vi "Generate SystemLink Software Tab shortcut.vi"() -> ()   [LabVIEW 2017]
uses:
  <vilib>/Utility/sysdir.llb/System Directory Type.ctl
panel:
  out "error out":errorcluster
  out "server URL":string
  out "local system minion ID":string
  # "Run this VI (or corresponding built EXE) to generate a Desktop shortcut to the Local System's SystemLink Software tab. \n\nNote: Before running this VI (or EXE), make sure that the local system has already successfully connected to and been approved by a SystemLink Server."
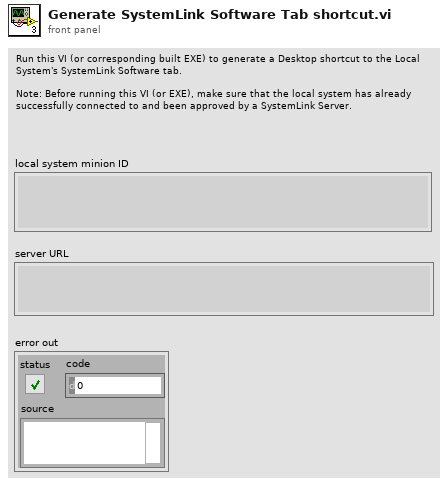
[diagram p1: front panel]
types:
  T1 = enum16{"open", "replace", "create", "open or create", "replace or create", "replace or create with confirmation"}
  T2 = typedef "System Directory Type.ctl" = i32
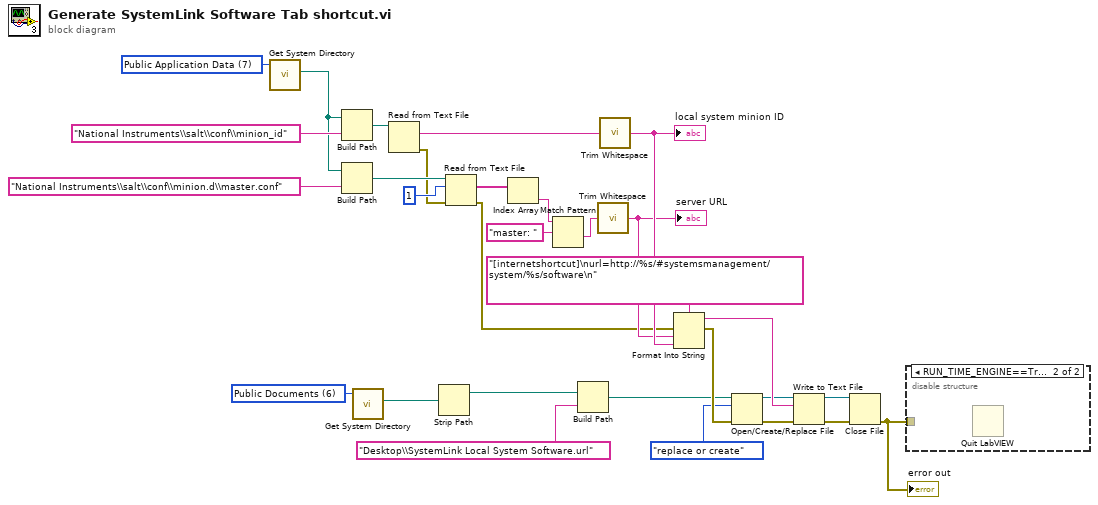
[diagram p0: block diagram]
diagram:
  w26 = T2 7 items=["User Home"=0, "User Desktop"=1, "User Documents"=2, "User Application Data"=3, "User Preferences"=4, "User Temporary"=5, "Public Documents"=6, "Public Application Data"=7, "Public Preferences"=8, "Public Cache"=13, "System Core Libraries"=9, "System Installed Libraries"=10, "Application Files"=11, "Boot Volume Root"=12] ("system directory type")
  w30 = T2 6 items=["User Home"=0, "User Desktop"=1, "User Documents"=2, "User Application Data"=3, "User Preferences"=4, "User Temporary"=5, "Public Documents"=6, "Public Application Data"=7, "Public Preferences"=8, "Public Cache"=13, "System Core Libraries"=9, "System Installed Libraries"=10, "Application Files"=11, "Boot Volume Root"=12] ("system directory type")
  n1 = call <vilib>:"Get System Directory.vi"("system directory type"=w26) -> ("system directory"=w21:path)  [unwired: 10 in]
  n2 = Build Path(base path=w21, name or relative path="National Instruments\\salt\\conf\\minion_id") -> (appended path=w24:path)
  n3 = Build Path(base path=w21, name or relative path="National Instruments\\salt\\conf\\minion.d\\master.conf") -> (appended path=w20:path)
  n4 = call <vilib>:"Get System Directory.vi"("system directory type"=w30) -> ("system directory"=w29:path)  [unwired: 10 in]
  n5 = Read from Text File(file (use dialog)=w24) -> (text=w23:string, error out=w7:errorcluster)  [unwired: 3 in, 2 out]
  n6 = Strip Path(path=w29) -> (stripped path=w28:path)  [unwired: 1 out]
  n7 = Read from Text File(file (use dialog)=w20, count=1, error in=w7) -> (text=w17:string[], error out=w6:errorcluster)  [unwired: 1 in, 2 out]
  n8 = Index Array(array=w17) -> (element=w16:string)  [unwired: 1 in]
  n9 = Match Pattern(string=w16, regular expression="master: ") -> (after substring=w14:string)  [unwired: 1 in, 3 out]
  n10 = Build Path(base path=w28, name or relative path="Desktop\\SystemLink Local System Software.url") -> (appended path=w3:path)
  n11 = call <vilib>:"Trim Whitespace.vi"("string"=w14) -> ("trimmed string"=w13:string)  [unwired: 1 in]
  "server URL" <- w13
  n12 = call <vilib>:"Trim Whitespace.vi"("string"=w23) -> ("trimmed string"=w19:string)  [unwired: 1 in]
  "local system minion ID" <- w19
  n13 = Format Into String(format string="[internetshortcut]\nurl=http://%s/#systemsmanagement/system/%s/software\n" ("name or relative path"), error in=w6, w13, w19) -> (resulting string=w11:string, error out=w5:errorcluster)  [unwired: 1 in]
  n14 = Open/Create/Replace File(file path (use dialog)=w3, error in=w5, operation (0:open)=T1."replace or create") -> (refnum out=w2:refnum<file>, error out=w4:errorcluster)  [unwired: 3 in, 1 out]
  n15 = Write to Text File(file (use dialog)=w2, text=w11, error in=w4) -> (refnum out=w10:refnum<file>, error out=w9:errorcluster)  [unwired: 1 in, 1 out]
  n16 = Close File(refnum=w10, error in=w9) -> (error out=w8:errorcluster)  [unwired: 1 out]
  "error out" <- w8
  n17 = disable-structure shown="RUN_TIME_ENGINE==True" {
    disable-tunnel: w8 -> [_ _]
    frame condition #0 (active) {
    }
    frame condition #1 {
      n18 = Quit LabVIEW() -> ()  [unwired: 1 in]
    }
  }
